vi "Run.vi"(8 "error in (no error)":errorcluster, 11 "API":T1) -> (0 "error out":errorcluster, 3 "API dup":T1)   [LabVIEW 2021, in "smo.lvlib" / "SMOFacade.lvclass"]
uses:
  SMOFacade.lvclass
  Registry/SMO_API--Cluster.ctl
  Terminal/Terminal.lvclass
  SMOFacade.lvclass/SMOFacade.ctl
  Registry/Registry-SMO.lvclass
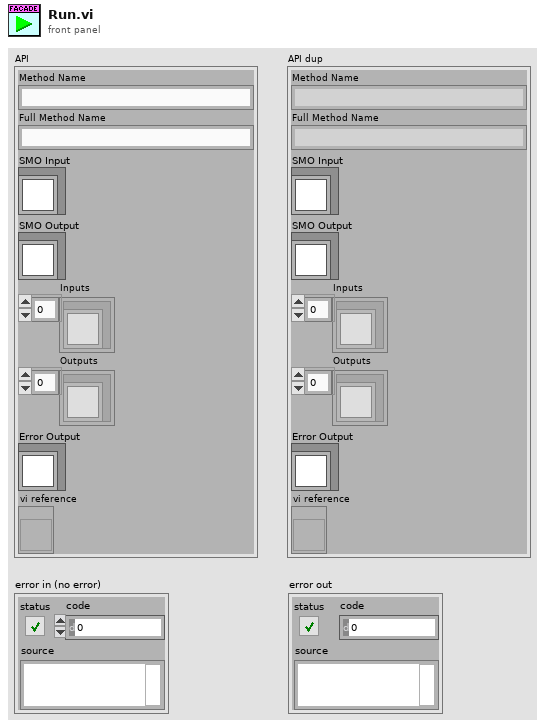
[diagram p1: front panel]
types:
  T1 = typedef "smo.lvlib/Registry-SMO.lvclass/SMO_API--Cluster.ctl" = cluster{"Method Name":string, "Full Method Name":string, "SMO Input":refnum<class "Terminal.lvclass">, "SMO Output":refnum<class "Terminal.lvclass">, "Inputs":refnum<class "Terminal.lvclass">[], "Outputs":refnum<class "Terminal.lvclass">[], "Error Output":refnum<class "Terminal.lvclass">, "vi reference":refnum<vi>}
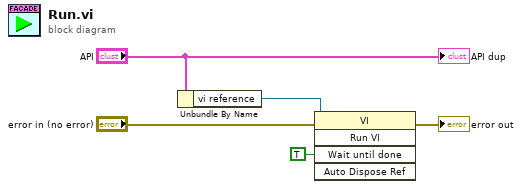
[diagram p0: block diagram]
diagram:
  n1 = Unbundle By Name("API") -> ("vi reference"=w2:refnum<vi>)
  n2 = invoke class="VI" method="Run VI"(reference=w2, error in="error in (no error)", "Wait until done"=TRUE ("Wait Until Done")) -> (error out=→"error out":errorcluster)  [unwired: 2 in, 4 out]
  "API dup" <- "API"
